vi "CSM-TagDBDisplayWnd.vi"(7 "Name(\"\" to use uuid)":string="UI.Exp.Template") -> ()   [LabVIEW 2020, in "CSM-TagDBDisplayWnd.lvlib"]
doc: "------------- lvcsm -------------\n[CSMStates]\nItem 0 = \"Idle\"\nItem 1 = \"CSM Documentation\"\nItem 2 = \"VI Reference\"\nItem 3 = \"Error Handler\"\nItem 4 = \"Critical Error\"\nItem 5 = \"Target Timeout Error\"\nItem 6 = \"Target Error\"\nItem 7 = \"Async Response\"\nItem 8 = \"Response\"\nItem 9 = \"Async Message Posted\"\nItem 10 = \"Initialize Core Data\"\nItem 11 = \"Exit\"\nItem 12 = \"Data: Initialize\"\nItem 13 = \"Data: Update Indicators\"\nItem 14 = \"Data: Load Attributes\"\nItem 15 = \"Data: Save Attributes\"\nItem 16 = \"Data: Cleanup\"\nItem 17 = \"Macro: Initialize\"\nItem 18 = \"Macro: Exit\"\nItem 19 = \"API: Start Refreshing\"\nItem 20 = \"API: Stop Refreshing\"\nItem 21 = \"Action: Insert TestStandOI\"\nItem 22 = \"Action: Relocate Boolean Switchs\"\nItem 23 = \"Action: Refresh Check\"\n\n[CSMStatus]\nItem 0 = \"Error Occurred@Error Handler\""
uses:
  CSM-TagDBDisplayWnd.lvlib
  a2febdbb-fb03-4ba6-9898-8a5d1d02332c.vi
  254342f9-cc88-4ec7-9cbe-7727ec765c53.vi
  d50deaec-bb00-4691-9d91-a2e409c005f3.vi
  1aa7de20-dba2-4569-9d21-b3d571cae75a.vi
  cbb8679f-6fca-4dfa-96de-e02d92bb6012.vi
  <userlib>/_NEVSTOP/Communicable State Machine(CSM)/AdvanceAPI/CSM - Revert Arguments-Safe String.vi
  <userlib>/_NEVSTOP/Communicable State Machine(CSM)/_Shared/Trim Single-line Text.vi
  <userlib>/_NEVSTOP/Communicable State Machine(CSM)/AdvanceAPI/CSM - Make String Arguments Safe.vi
  <userlib>/_NEVSTOP/Communicable State Machine(CSM)/AdvanceAPI/CSM - Break Down Multiple States String.vi
  <userlib>/_NEVSTOP/Communicable State Machine(CSM)/AdvanceAPI/CSM - Compact Multiple States.vi
  a2febdbb-fb03-4ba6-9898-8a5d1d02332c.vi/99de0c97-112a-4c86-9094-c187659127e1.vi
  <userlib>/_NEVSTOP/Communicable State Machine(CSM)/Utility/Build Error Cluster.vi
  <userlib>/_NEVSTOP/Communicable State Machine(CSM)/AdvanceAPI/CSM - Convert HexStr to Data.vi
  <userlib>/_NEVSTOP/Communicable State Machine(CSM)/AdvanceAPI/CSM - Keywords.vi
  <userlib>/_NEVSTOP/Communicable State Machine(CSM)/_Polymophic/CSM - Filter Duplicated Lines.vi
  <vilib>/Utility/Data Type/Get Type Information.vi
  <userlib>/_NEVSTOP/Communicable State Machine(CSM)/addons/API-String-Arugments-Support/_Support/Data To SingleElementsArray_csm.vi
  <userlib>/_NEVSTOP/Communicable State Machine(CSM)/addons/API-String-Arugments-Support/_Support/Data To API String Arguments.vi
  <userlib>/_NEVSTOP/Communicable State Machine(CSM)/addons/INI-Static-Variable-Support/_Support/Parse Used Session and Name.vi
  <userlib>/_NEVSTOP/Communicable State Machine(CSM)/addons/INI-Static-Variable-Support/_Support/INI-FGV(lvlibp).vi
  <userlib>/_NEVSTOP/Communicable State Machine(CSM)/addons/INI-Static-Variable-Support/_Support/Populate String with INI Variable.vi
  <userlib>/_NEVSTOP/Communicable State Machine(CSM)/addons/API-String-Arugments-Support/_Support/Convert API String Arguments to Data(variant).vi
  <userlib>/_NEVSTOP/Communicable State Machine(CSM)/addons/API-String-Arugments-Support/_Support/SingleElementsArray To Data_csm.vi
  <userlib>/_NEVSTOP/TagDB/Add-ons/RefManager/_Support/UISync/_Pull Controls Value to DPs(VI).vi
  <userlib>/_NEVSTOP/TagDB/Add-ons/RefManager/_Support/UISync/_Publish DP Indicators(VI).vi
  DefaultPage.vi
  <userlib>/_NEVSTOP/Communicable State Machine(CSM)/Communicable State Machine.lvlib
  <userlib>/_NEVSTOP/Communicable State Machine(CSM)/addons/Logger/CSM File Logger.lvlib
  <userlib>/_NEVSTOP/Communicable State Machine(CSM)/addons/Loop-Support/CSM Loop Support.lvlib
  <userlib>/_NEVSTOP/Communicable State Machine(CSM)/addons/INI-Static-Variable-Support/INI-Static-Variable-Support.lvlib
  <userlib>/_NEVSTOP/TagDB/TagDB.lvlib
  <userlib>/_NEVSTOP/TagDB/Add-ons/RefManager/TagDB RefManager.lvlib
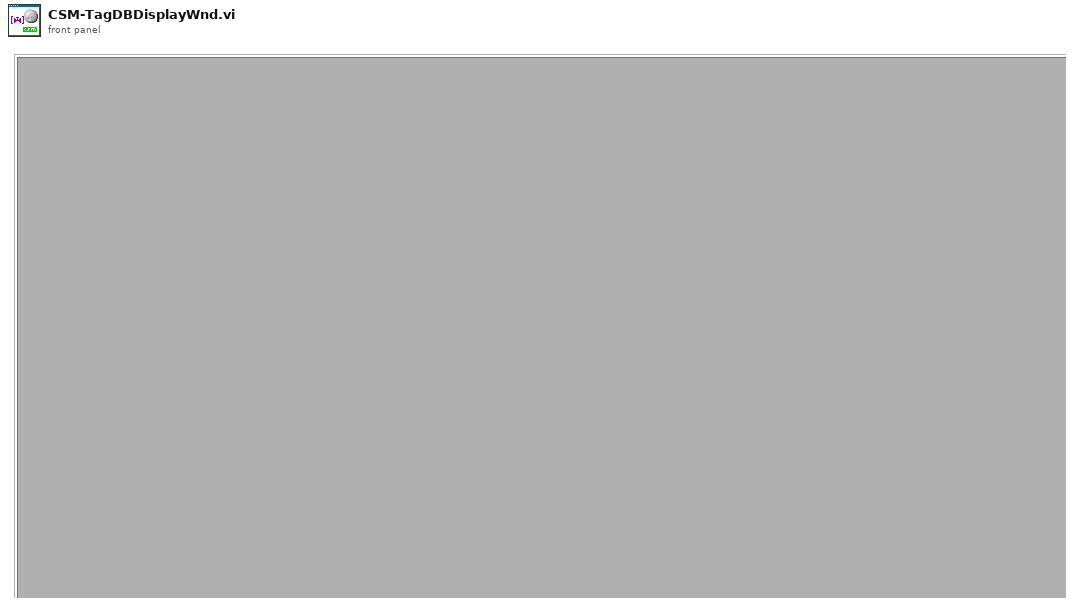
[diagram p1: front panel]
types:
  T1 = enum32{"Invalid", "Standard", "Closed", "Hidden", "Minimized", "Maximized"}
  T2 = enum32{"invalid app kind", "Development System", "Run Time System", "Student Edition", "Embedded LabVIEW", "Evaluation", "Custom"}
  T3 = typedef "Communicable State Machine.lvlib/_CSM_Response Source Message.ctl" = cluster{"‘State":string, "’Arguments":string, "’Error":errorcluster}
  T4 = cluster{"Current VI Reference":refnum<vi>, "Close Panel on Exit?":bool}
  T5 = cluster{"Core":cluster{"Current VI Reference":refnum<vi>, "Close Panel on Exit?":bool}, "SearchingPath":path[], "PageRef":refnum<vi>, "DefaultPage":string}
  T6 = cluster{"SearchingPath":path[], "DefaultPage":string}
  T7 = enum32{"Bad", "Idle", "Run top level", "Running"}
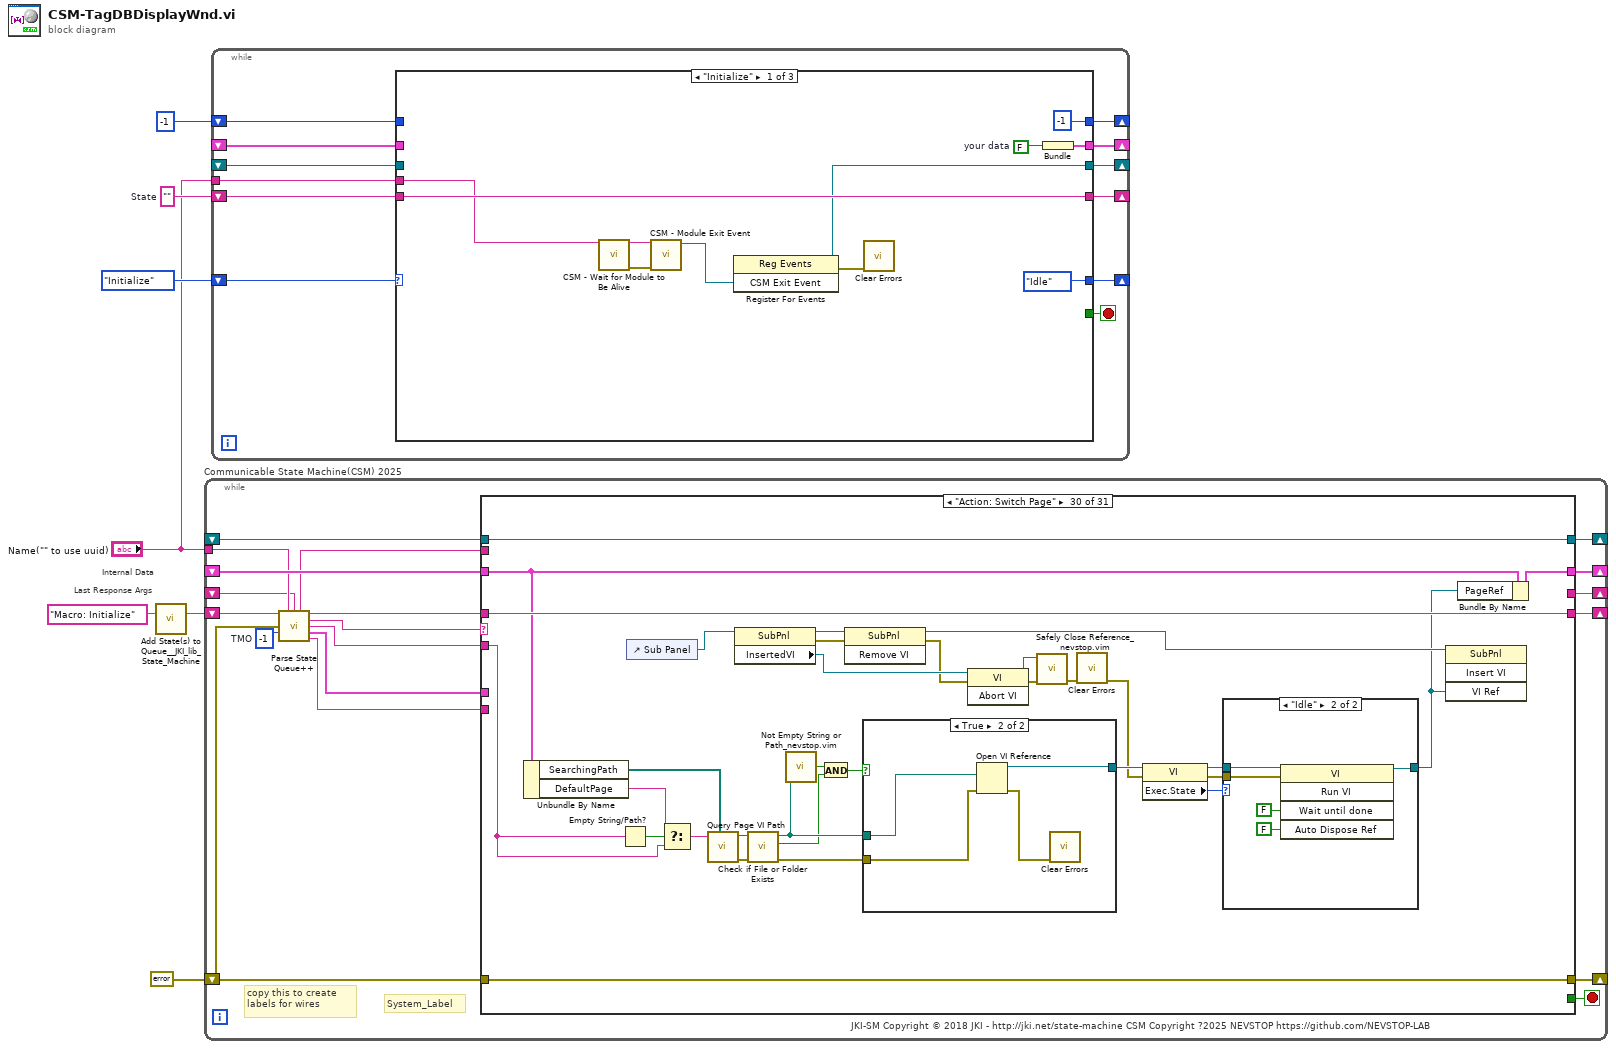
[diagram p0: block diagram]
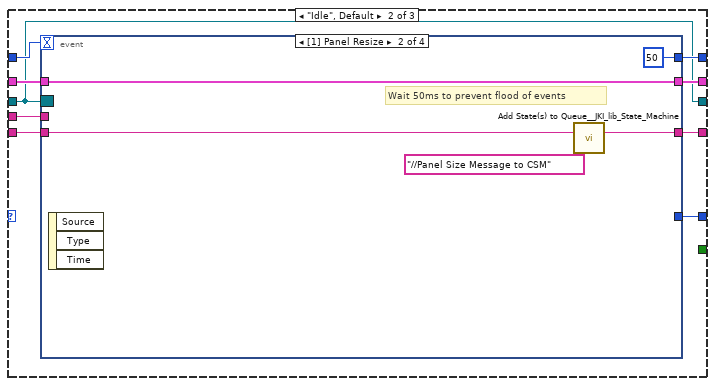
[diagram p2: hidden frame]
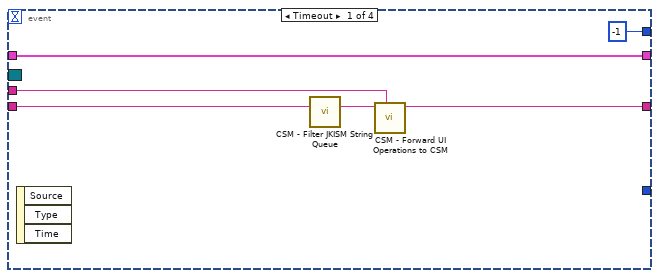
[diagram p3: hidden frame]
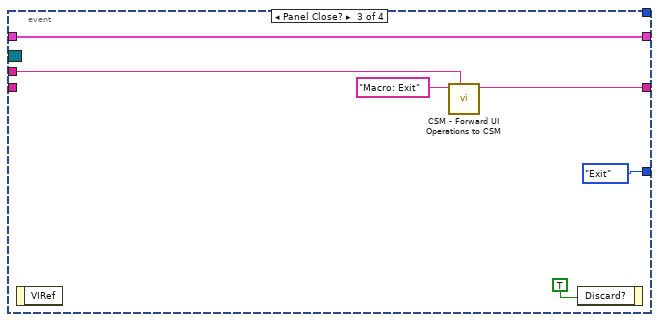
[diagram p4: hidden frame]
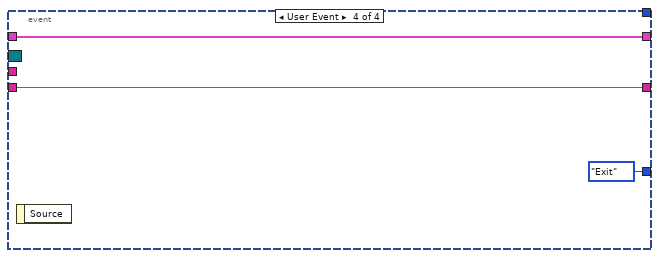
[diagram p5: hidden frame]
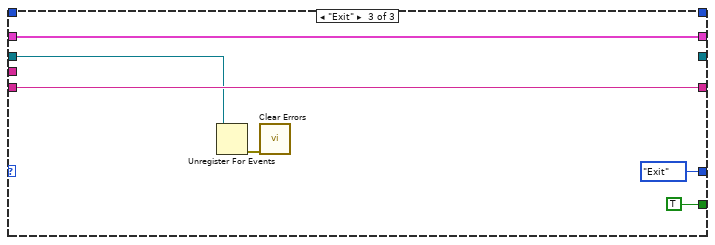
[diagram p6: hidden frame]
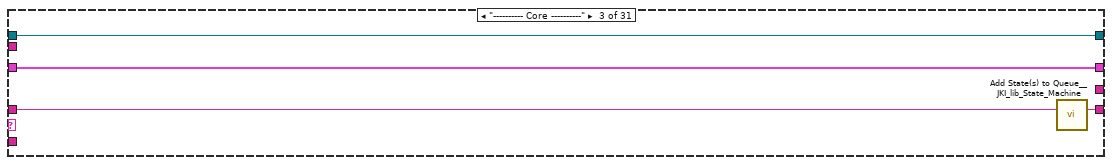
[diagram p9: hidden frame]
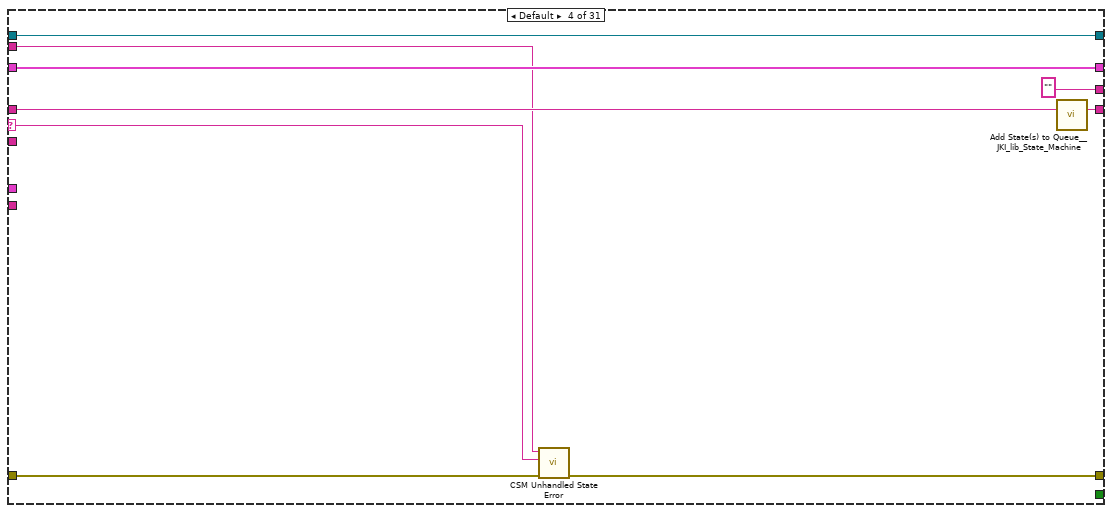
[diagram p10: hidden frame]
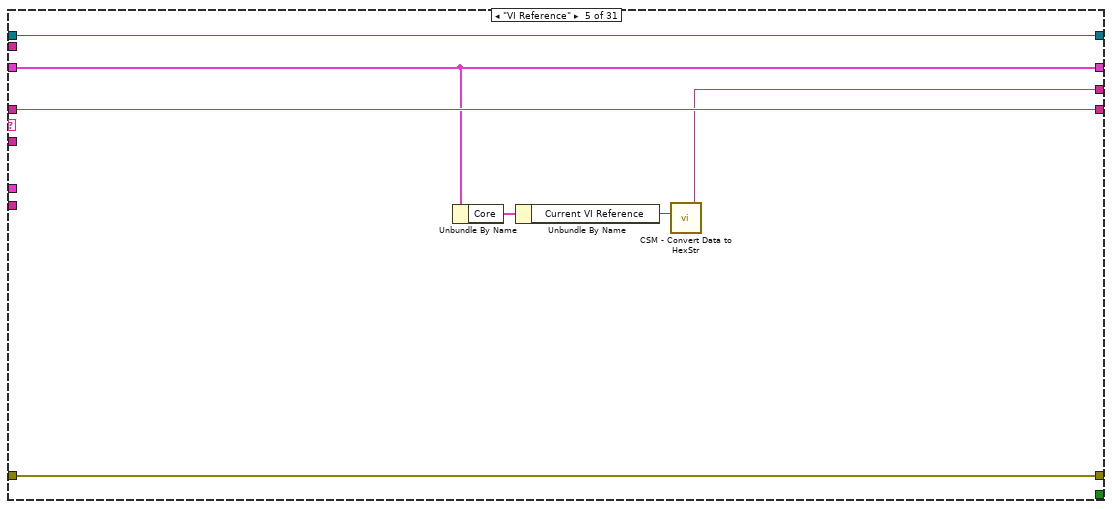
[diagram p11: hidden frame]
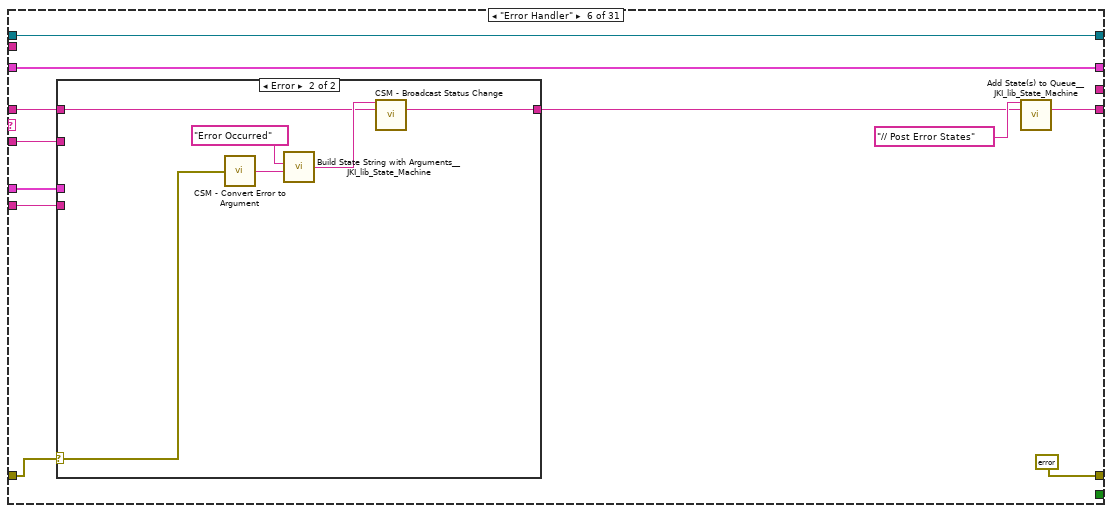
[diagram p12: hidden frame]
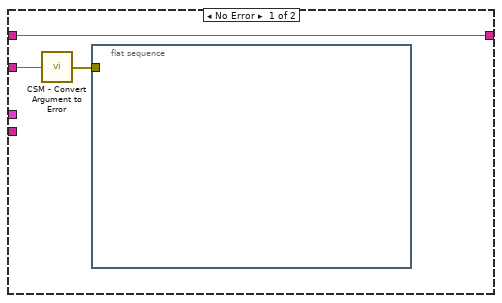
[diagram p13: hidden frame]
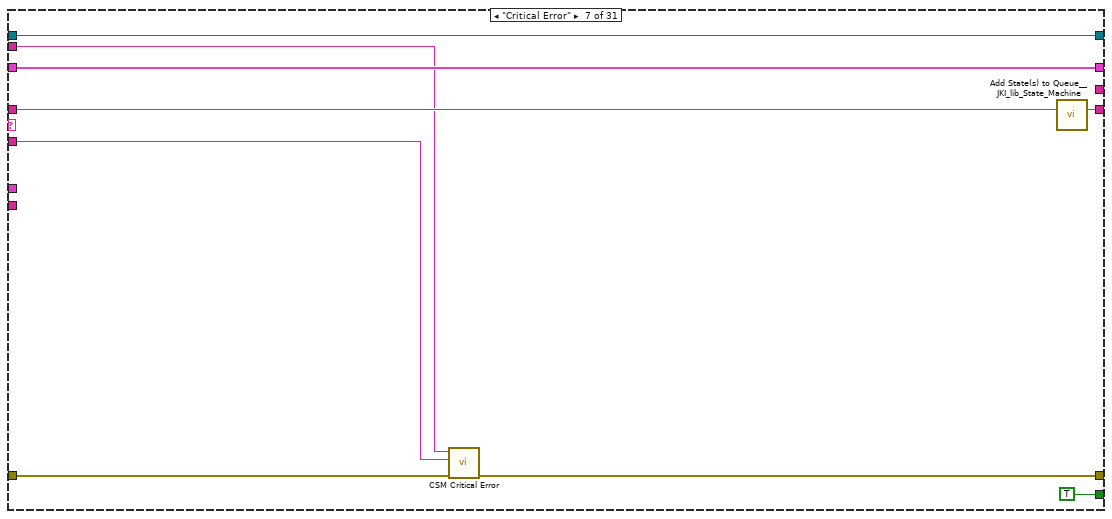
[diagram p14: hidden frame]
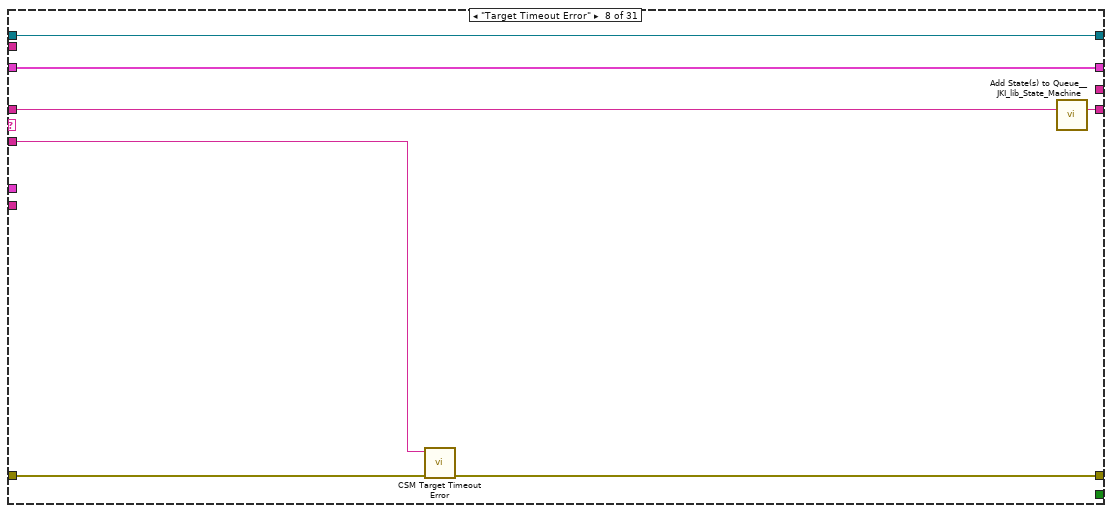
[diagram p15: hidden frame]
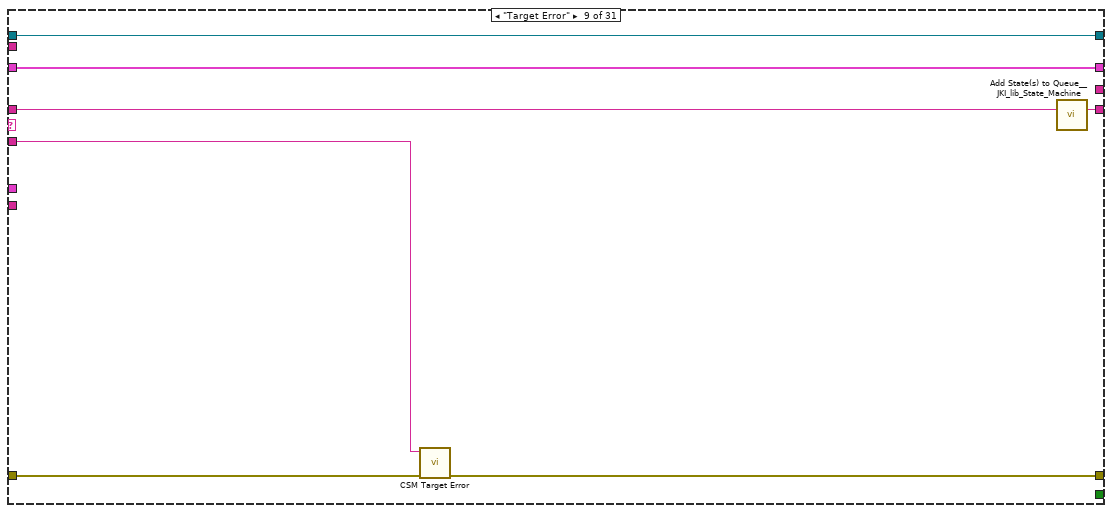
[diagram p16: hidden frame]
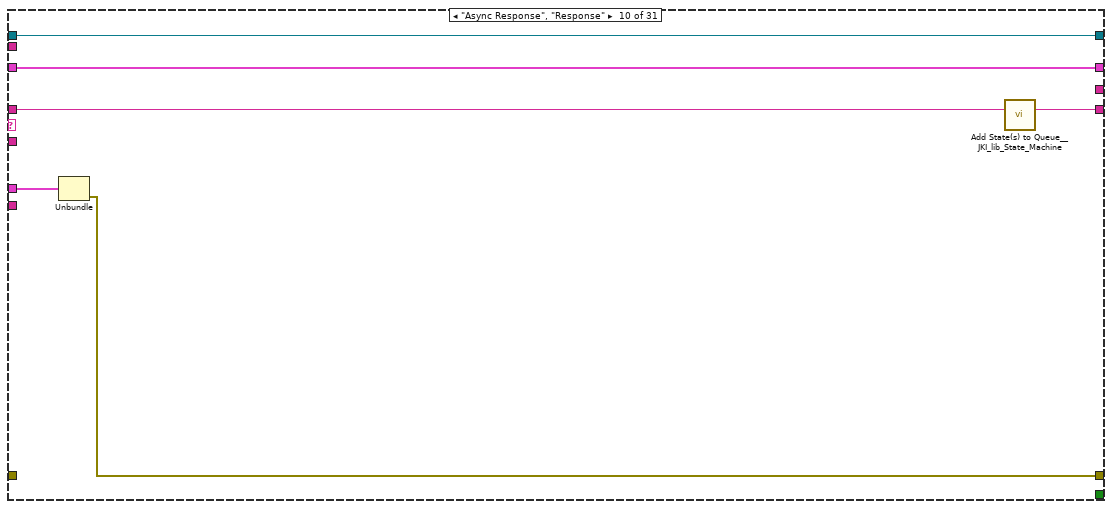
[diagram p17: hidden frame]
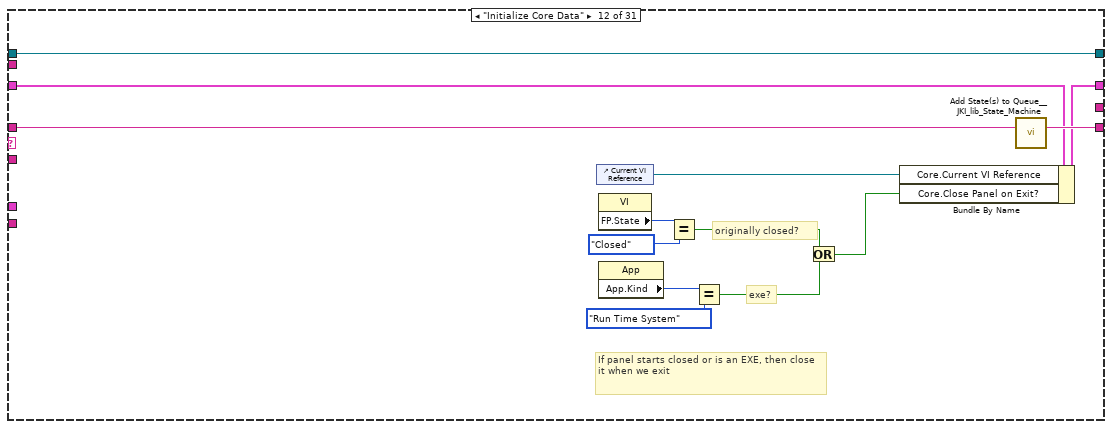
[diagram p19: hidden frame]
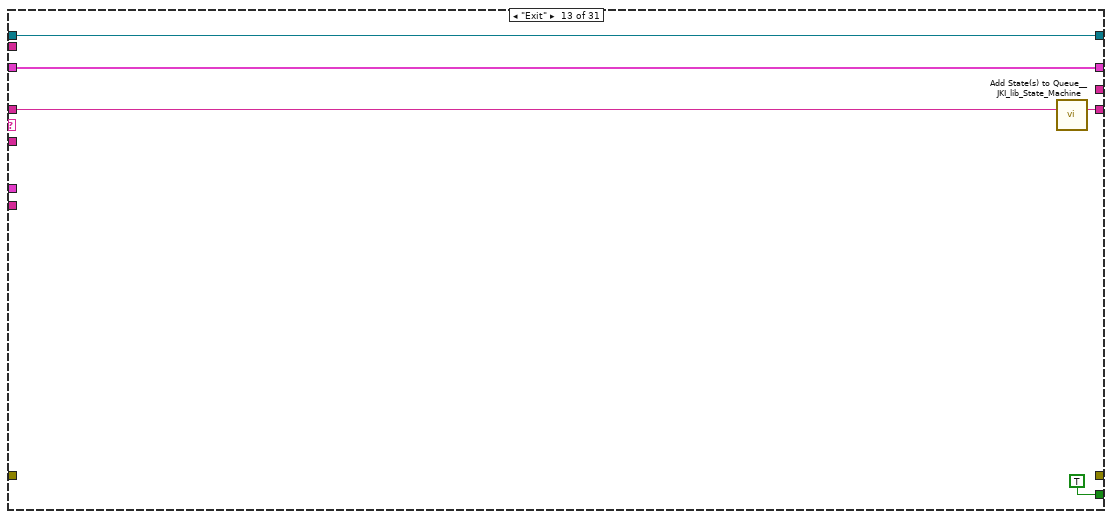
[diagram p20: hidden frame]
diagram:
  w3 = ""  # State
  # "Last Response Args"
  # "Internal Data"
  n1 = call <vilib>:"Add State(s) to Queue__JKI_lib_State_Machine.vi"("State(s) in (\"\")"="Macro: Initialize" ("Init State(\"Macro: Initialize\")")) -> ("States Out"=w7:string)  [unwired: 14 in]
  n2 = while "Communicable State Machine(CSM) 2025" {
    shift-right: [w21] -> _
    shift-left: _ -> [w20]
    shift-right: [w24] -> _
    shift-left: errorcluster {"status"=FALSE, "code"=0, "source"=""} ("error out") -> [w10]
    shift-right: [w23] -> _
    shift-left: w7 -> [w25]
    tunnel: "Name(\"\" to use uuid)" -> [w17]
    shift-right: [w18] -> _
    shift-left: _ -> [w12]
    shift-right: [w9] -> _
    shift-left: _ -> [w8]
    stop <- w22 stop-if-true
    w19 = -1  # TMO
    # "JKI-SM Copyright © 2018 JKI - http://jki.net/state-machine CSM Copyright ?2025 NEVSTOP https://github.com/NEVSTOP-LAB"
    # "copy this to create labels for wires"
    # "System_Label"
    n3 = call <userlib>:"Parse State Queue++.vi"("State Queue"=w25, "Name (\"\" to Use UUID)"=w17, "Response Arguments"=w12, "Previous Error"=w10, "Dequeue (1 ms)"=w19) -> ("Name Used"=w11:string, "Remaining States"=w26:string, "Current State"=w13:string, "Arguments"=w14:string, "Additional Information"=w15:T3, "Source CSM"=w16:string)  [unwired: 5 in]
    n4 = case shown="\"Action: Switch Page\"" w13 {
      selector: w13 -> [_ _ _ w41 _ _ _ _ _ _ _ _ _ _ _ _ _ _ _ _ _ _ _ _ _ _ _ _ _ _ w289]
      tunnel: w26 -> [w28 w32 w36 w45 w51 w57 w81 w88 w95 w101 w104 w117 w122 w126 w147 w150 w153 w156 w171 w175 w180 w187 w190 w198 w209 w216 w222 w226 w235 w275 w292]
      tunnel: w14 -> [_ _ _ _ _ w56 w77 w85 w92 _ _ _ _ _ _ _ _ _ _ _ _ _ _ w193 w206 _ _ _ _ w262 _]
      tunnel: w20 -> [w29 w31 w34 w43 w50 w62 w79 w86 w93 w99 w103 w111 w120 w124 _ w149 w152 w155 w166 w173 w178 w185 w189 w197 w212 w218 w221 w224 w232 w269 w294]
      tunnel: [_ _ _ w38 w52 errorcluster {"status"=FALSE, "code"=0, "source"=""} ("error out") w74 w83 w90 w97 _ _ _ _ w133 _ _ _ w167 _ _ _ _ w194 w213 _ _ _ w227 w276 w295] -> w24
      tunnel: w10 -> [_ _ _ w39 w52 w60 w75 w84 w91 _ _ _ _ _ _ _ _ _ w168 _ _ _ _ _ w213 _ _ _ w228 w276 w295]
      tunnel: [w28 w32 w35 w44 w51 w58 w80 w87 w94 w100 w104 w116 w121 w125 w146 w150 w153 w156 w170 w174 w179 w186 w190 w198 w210 w215 w219 w225 w235 w275 w291] -> w23
      tunnel: [_ _ _ _ _ _ TRUE _ _ _ _ _ TRUE _ _ _ _ _ _ _ _ _ _ _ _ _ _ _ _ _ _] -> w22
      tunnel: [w29 w31 w34 w43 w50 w62 w79 w86 w93 w99 w103 w115 w120 w124 w138 w149 w152 w155 w166 w173 w178 w185 w189 w197 w212 w218 w221 w224 w232 w246 w294] -> w21
      tunnel: w16 -> [_ _ _ _ _ w55 _ _ _ _ _ _ _ _ _ _ _ _ _ _ _ _ _ _ _ _ _ _ _ _ _]
      tunnel: w15 -> [_ _ _ _ _ w54 _ _ _ w98 _ _ _ _ _ _ _ _ _ _ _ _ _ _ _ _ _ _ _ _ _]
      tunnel: [_ _ _ "" w47 _ _ _ _ _ _ _ _ _ _ _ _ _ _ _ _ _ _ _ _ _ _ _ _ _ _] -> w18
      tunnel: w11 -> [_ _ _ w40 _ _ w76 _ _ _ _ _ _ _ w140 _ _ _ _ _ _ _ _ _ _ _ _ _ _ _ _]
      tunnel: [w27 w30 w33 w37 w46 w53 w73 w82 w89 w96 w102 w105 w118 w123 refnum<k1> refnum ("TagDB") w148 w151 w154 w165 w172 w176 w181 w188 w195 w211 w217 w220 w223 w233 w274 w293] -> w9
      tunnel: w8 -> [w27 w30 w33 w37 w46 w53 w73 w82 w89 w96 w102 w105 w118 w123 _ w148 w151 w154 w165 w172 w176 w181 w188 w196 w211 w217 w220 w223 w234 w274 w293]
      frame "", "Idle" {
      }
      frame "CSM Documentation" {
      }
      frame "---------- Core ----------" {
        n5 = call <vilib>:"Add State(s) to Queue__JKI_lib_State_Machine.vi"("State(s) in (\"\")"=w36) -> ("States Out"=w35:string)  [unwired: 14 in]
      }
      frame Default {
        n6 = call <userlib>:"CSM Unhandled State Error.vi"("error in (no error)"=w39, "Undefined State"=w41, "CSM Name"=w40) -> ("error out"=w38:errorcluster)  [unwired: 8 in]
        n7 = call <vilib>:"Add State(s) to Queue__JKI_lib_State_Machine.vi"("State(s) in (\"\")"=w45) -> ("States Out"=w44:string)  [unwired: 14 in]
      }
      frame "VI Reference" {
        n8 = Unbundle By Name(w50) -> ("Core"=w49:T4)
        n9 = Unbundle By Name(w49) -> ("Current VI Reference"=w48:refnum<vi>)
        n10 = call <userlib>:"CSM - Convert Data to HexStr.vi"("Variant"=w48) -> ("HEX String (0-9,A-F)"=w47:string)  [unwired: 8 in]
      }
      frame "Error Handler" {
        n11 = case shown="Error" w60 {
          selector: w60 -> [_ w67]
          tunnel: [w66 w69] -> w59
          tunnel: w57 -> [w66 w68]
          tunnel: w56 -> [w65 _]
          tunnel: w55 -> [_ _]
          tunnel: w54 -> [_ _]
          frame No Error {
            n12 = call <userlib>:"CSM - Convert Argument to Error.vi"("Argument"=w65) -> ("Error"=w64:errorcluster)  [unwired: 4 in]
            n13 = flat-sequence {
              tunnel: w64 -> [_]
              frame #0 {
              }
            }
          }
          frame Error {
            n14 = call <userlib>:"CSM - Convert Error to Argument.vi"("Error"=w67) -> ("Argument"=w71:string)  [unwired: 4 in]
            n15 = call <vilib>:"Build State String with Arguments__JKI_lib_State_Machine.vi"("Arguments (\"\")"=w71, "State"="Error Occurred" ("Status with Arguments")) -> ("State with Arguments"=w70:string)  [unwired: 4 in]
            n16 = call <userlib>:"CSM - Broadcast Status Change.vi"("Status With Arguments"=w70, "State Queue"=w68) -> ("Remaining States"=w69:string)  [unwired: 13 in]
          }
        }
        n17 = call <vilib>:"Add State(s) to Queue__JKI_lib_State_Machine.vi"("State(s) in Front (\"\")"="// Post Error States", "State(s) in (\"\")"=w59) -> ("States Out"=w58:string)  [unwired: 13 in]
      }
      frame "Critical Error" {
        n18 = call <userlib>:"CSM Critical Error.vi"("error in (no error)"=w75, "Arugments (As Reason)"=w77, "CSM Name"=w76) -> ("error out"=w74:errorcluster)  [unwired: 8 in]
        n19 = call <vilib>:"Add State(s) to Queue__JKI_lib_State_Machine.vi"("State(s) in (\"\")"=w81) -> ("States Out"=w80:string)  [unwired: 14 in]
      }
      frame "Target Timeout Error" {
        n20 = call <userlib>:"CSM Target Timeout Error.vi"("error in (no error)"=w84, "Arguments (As CSM Name)"=w85) -> ("error out"=w83:errorcluster)  [unwired: 9 in]
        n21 = call <vilib>:"Add State(s) to Queue__JKI_lib_State_Machine.vi"("State(s) in (\"\")"=w88) -> ("States Out"=w87:string)  [unwired: 14 in]
      }
      frame "Target Error" {
        n22 = call <userlib>:"CSM Target Error.vi"("error in (no error)"=w91, "Arguments (As CSM Name)"=w92) -> ("error out"=w90:errorcluster)  [unwired: 9 in]
        n23 = call <vilib>:"Add State(s) to Queue__JKI_lib_State_Machine.vi"("State(s) in (\"\")"=w95) -> ("States Out"=w94:string)  [unwired: 14 in]
      }
      frame "Async Response", "Response" {
        n24 = Unbundle(w98) -> ("’Error"=w97:errorcluster)  [unwired: 2 out]
        n25 = call <vilib>:"Add State(s) to Queue__JKI_lib_State_Machine.vi"("State(s) in (\"\")"=w101) -> ("States Out"=w100:string)  [unwired: 14 in]
      }
      frame "Async Message Posted" {
      }
      frame "Initialize Core Data" {
        # "originally closed?"
        # "exe?"
        # "If panel starts closed or is an EXE, then close it when we exit"
        n26 = control-ref of="Current VI Reference"() -> (w109:refnum<vi>)
        n27 = property class="VI"() -> ("FP.State"=w108:T1)  [unwired: 2 in, 2 out]
        n28 = property class="App"() -> ("App.Kind"=w114:T2)  [unwired: 2 in, 2 out]
        n29 = Equal?(x=w108, y=T1."Closed" ("Front Panel Window:State")) -> (x = y?=w106:bool)
        n30 = Equal?(x=w114, y=T2."Run Time System" ("Application:Kind")) -> (x = y?=w112:bool)
        n31 = Or(x=w106, y=w112) -> (x .or. y?=w110:bool)
        n32 = Bundle By Name(cluster=w111, "Core.Current VI Reference"=w109, "Core.Close Panel on Exit?"=w110) -> (w115:T5)
        n33 = call <vilib>:"Add State(s) to Queue__JKI_lib_State_Machine.vi"("State(s) in (\"\")"=w117) -> ("States Out"=w116:string)  [unwired: 14 in]
      }
      frame "Exit" {
        n34 = call <vilib>:"Add State(s) to Queue__JKI_lib_State_Machine.vi"("State(s) in (\"\")"=w122) -> ("States Out"=w121:string)  [unwired: 14 in]
      }
      frame "---------- Data ----------" {
        n35 = call <vilib>:"Add State(s) to Queue__JKI_lib_State_Machine.vi"("State(s) in (\"\")"=w126) -> ("States Out"=w125:string)  [unwired: 14 in]
      }
      frame "Data: Initialize" {
        w127 = "*"  # DefaultPage
        w137 = ""  # DefaultPage
        w142 = refnum<vi> refnum  # PageRef
        w139 = path[] []  # SearchingPath
        w144 = T4 {"Current VI Reference"=refnum, "Close Panel on Exit?"=FALSE}  # Core
        n36 = Bundle("Core"=w144, "SearchingPath"=w139, "PageRef"=w142, "DefaultPage"=w137) -> (w145:T5)  [unwired: 1 in]
        n37 = Bundle("SearchingPath"=w139, "DefaultPage"=w137) -> (w141:T6)  [unwired: 1 in]
        n38 = call "CSM - Read Cluster Elements From Session.vim"("Section Name (\"\" as Default)"=w140, "Cluster"=w141) -> ("error out"=w133:errorcluster, "Cluster out"=w136:T6)  [unwired: 6 in]
        n39 = Unbundle By Name(w136) -> ("SearchingPath"=w135:path[], "DefaultPage"=w134:string)
        n40 = call <userlib>:"CSM Application Directory.vi"() -> ("CSM Application Dir"=w128:path)  [unwired: 11 in]
        n41 = Current VI's Path() -> (path=w131:path)
        n42 = Build Path(base path=w128, name or relative path=w127) -> (appended path=w129:path)
        n43 = call <userlib>:"First Existing Folder in Path.vi"("Stripped Path In"=w131) -> ("Stripped Path Out"=w130:path)  [unwired: 10 in]
        n44 = Build Array (concatenate)(w135, w130, w129) -> (w132:path[])
        n45 = Bundle By Name(cluster=w145, "SearchingPath"=w132, "DefaultPage"=w134) -> (w138:T5)
        n46 = call <vilib>:"Add State(s) to Queue__JKI_lib_State_Machine.vi"("State(s) in (\"\")"=w147) -> ("States Out"=w146:string)  [unwired: 14 in]
      }
      frame "Data: Update Indicators" {
      }
      frame "Data: Load Attributes" {
      }
      frame "Data: Save Attributes" {
      }
      frame "Data: Cleanup" {
        n47 = Unbundle By Name(w166) -> ("Core.Current VI Reference"=w169:refnum<vi>)
        n48 = control-ref of="Sub Panel"() -> (w164:refnum<vi>)
        n49 = property class="SubPnl"(reference=w164) -> (reference out=w158:refnum<vi>, error out=w159:errorcluster, "InsertedVI"=w163:refnum<vi>)  [unwired: 1 in]
        n50 = invoke class="SubPnl" method="Remove VI"(reference=w158, error in=w159) -> (error out=w157:errorcluster)  [unwired: 1 in, 2 out]
        n51 = Close Reference(reference=w169, error in (no error)=w168) -> (error out=w167:errorcluster)
        n52 = invoke class="VI" method="Abort VI"(reference=w163, error in=w157) -> (reference out=w161:refnum<vi>, error out=w162:errorcluster)  [unwired: 1 in, 1 out]
        n53 = call "Safely Close Reference_nevstop.vim"("error in (no error)"=w162, "Reference"=w161) -> ("error out"=w160:errorcluster)  [unwired: 9 in]
        n54 = call <vilib>:"Clear Errors.vi"("error in (no error)"=w160) -> ()  [unwired: 5 in, 2 out]
        n55 = call <vilib>:"Add State(s) to Queue__JKI_lib_State_Machine.vi"("State(s) in (\"\")"=w171) -> ("States Out"=w170:string)  [unwired: 14 in]
      }
      frame "---------- Macro ----------" {
        n56 = call <vilib>:"Add State(s) to Queue__JKI_lib_State_Machine.vi"("State(s) in (\"\")"=w175) -> ("States Out"=w174:string)  [unwired: 14 in]
      }
      frame "Macro: Initialize" {
        n57 = call <vilib>:"Add State(s) to Queue__JKI_lib_State_Machine.vi"("State(s) in Front (\"\")"="Data: Initialize\nData: Load Attributes\nInitialize Core Data\nData: Update Indicators\nAction: Switch Page\nAPI: Start", "State(s) in (\"\")"=w180) -> ("States Out"=w179:string)  [unwired: 13 in]
      }
      frame "Macro: Exit" {
        n58 = call <vilib>:"Add State(s) to Queue__JKI_lib_State_Machine.vi"("State(s) in Front (\"\")"="//Exit Sub-Modules ", "State(s) at Back (\"\")"="Data: Save Attributes\nData: Cleanup\nExit") -> ("States Out"=w183:string)  [unwired: 13 in]
        n59 = call <vilib>:"Add State(s) to Queue__JKI_lib_State_Machine.vi"("State(s) in Front (\"\")"=w183, "State(s) in (\"\")"=w187) -> ("States Out"=w186:string)  [unwired: 13 in]
      }
      frame "---------- API ----------" {
      }
      frame "API: Set TagDB" {
        n60 = call <userlib>:"Is HexStr Content.vi"("Content"=w193) -> ("hexStr"=w191:string, "HexStr Content"=w192:bool)  [unwired: 9 in]
        n61 = case shown="True" w192 {
          tunnel: w196 -> [_ w205]
          tunnel: [w201 w204] -> w195
          tunnel: [w200 w203] -> w194
          tunnel: w191 -> [w199 w202]
          frame False {
            n62 = call <userlib>:"TagDB-Obtain.vi"("name (unnamed)"=w199) -> ("error out"=w200:errorcluster, "TagDB"=w201:refnum<k1>)  [unwired: 4 in, 1 out]
          }
          frame True {
            n63 = call "CSM - Convert HexStr to Data.vim"("Type"=w205, "HEX String"=w202) -> ("Error out"=w203:errorcluster, "data"=w204:refnum<k1>)  [unwired: 6 in]
          }
        }
      }
      frame "API: Switch" {
        n64 = call <vilib>:"Build State String with Arguments__JKI_lib_State_Machine.vi"("Arguments (\"\")"=w206, "State"="Action: Switch Page") -> ("State with Arguments"=w207:string)  [unwired: 4 in]
        n65 = call <vilib>:"Add State(s) to Queue__jki_lib_state_machine.vi"("State(s) in Front (\"\")"=w207, "State(s) in (\"\")"=w209) -> ("States Out"=w210:string)  [unwired: 13 in]
      }
      frame "API: Start" {
        n66 = call <userlib>:"CSMLS - Define Loop State(s).vi"("Loop States"="Action: Loop Check -><loop>", "States Queue"=w216) -> ("Remaining States"=w215:string)  [unwired: 13 in]
      }
      frame "API: Stop" {
        n67 = call <userlib>:"CSMLS - Remove Loop Tag to Break.vi"("States Queue"=w222) -> ("Remaining States"=w219:string)  [unwired: 10 in]
      }
      frame "---------- Action ----------" {
        n68 = call <vilib>:"Add State(s) to Queue__JKI_lib_State_Machine.vi"("State(s) in (\"\")"=w226) -> ("States Out"=w225:string)  [unwired: 14 in]
      }
      frame "Action: Refresh TagDB Display" {
        n69 = Unbundle By Name(w232) -> ("PageRef"=w231:refnum<vi>)
        n70 = Not A Number/Path/Refnum?(number/path/refnum=w231) -> (NaN/Path/Refnum?=w229:bool)
        n71 = Not(x=w229) -> (.not. x?=w230:bool)
        n72 = case shown="True" w230 {
          tunnel: w234 -> [w237 w244]
          tunnel: [w237 w242] -> w233
          tunnel: w231 -> [_ w238]
          tunnel: w228 -> [w236 w239]
          tunnel: [w236 w241] -> w227
          frame False {
          }
          frame True {
            n73 = call-poly <userlib>:"Pull Controls Value to DPs.vi"("VIRef(Caller VI)"=w238, "error in (no error)"=w239, "SILAPI In"=w244) -> ("error out"=w240:errorcluster, "SILAPI Out"=w243:refnum<k1>)  [unwired: 6 in, 1 out]
            n74 = call-poly <userlib>:"Publish DP Indicators.vi"("VIRef(Caller VI)/RefMgr"=w238, "error in (no error)"=w240, "SILAPI In"=w243) -> ("error out"=w241:errorcluster, "SILAPI Out"=w242:refnum<k1>)  [unwired: 6 in, 1 out]
          }
        }
      }
      frame "Action: Switch Page" {
        n75 = Unbundle By Name(w269) -> ("SearchingPath"=w268:path[], "DefaultPage"=w263:string)
        n76 = Empty String/Path?(string/path=w262) -> (empty?=w264:bool)
        n77 = control-ref of="Sub Panel"() -> (w249:refnum<vi>)
        n78 = Select(t=w263, s=w264, f=w262) -> (s? t:f=w261:string)
        n79 = call "Query Page VI Path.vi"("searching path"=w268, "page name"=w261) -> ("Error out"=w266:errorcluster, "path"=w267:path)  [unwired: 8 in]
        n80 = property class="SubPnl"(reference=w249) -> (reference out=w251:refnum<vi>, error out=w252:errorcluster, "InsertedVI"=w256:refnum<vi>)  [unwired: 1 in]
        n81 = call <vilib>:"Check if File or Folder Exists.vi"("error in (no error)"=w266, "path"=w267) -> ("error out"=w265:errorcluster, "file or folder exists?"=w258:bool, "dup path"=w260:path)  [unwired: 7 in]
        n82 = call "Not Empty String or Path_nevstop.vim"("String"=w260) -> ("not empty?"=w259:bool)
        n83 = And(x=w259, y=w258) -> (x .and. y?=w257:bool)
        n84 = invoke class="SubPnl" method="Remove VI"(reference=w251, error in=w252) -> (reference out=w247:refnum<vi>, error out=w250:errorcluster)  [unwired: 1 in, 1 out]
        n85 = case shown="True" w257 {
          tunnel: [w277 w281] -> w273
          tunnel: w260 -> [_ w280]
          tunnel: w265 -> [_ w279]
          frame False {
            n86 = vi-ref "CSM-TagDBDisplayWnd.lvlib:DefaultPage.vi"() -> (w277:refnum<vi>)
          }
          frame True {
            n87 = Open VI Reference(vi path=w280, error in (no error)=w279) -> (vi reference=w281:refnum<vi>, error out=w278:errorcluster)  [unwired: 4 in]
            n88 = call <vilib>:"Clear Errors.vi"("error in (no error)"=w278) -> ()  [unwired: 5 in, 2 out]
          }
        }
        n89 = invoke class="VI" method="Abort VI"(reference=w256, error in=w250) -> (reference out=w254:refnum<vi>, error out=w255:errorcluster)  [unwired: 1 in, 1 out]
        n90 = call "Safely Close Reference_nevstop.vim"("error in (no error)"=w255, "Reference"=w254) -> ("error out"=w253:errorcluster)  [unwired: 9 in]
        n91 = call <vilib>:"Clear Errors.vi"("error in (no error)"=w253) -> ("error out"=w248:errorcluster)  [unwired: 5 in, 1 out]
        n92 = property class="VI"(reference=w273, error in=w248) -> (reference out=w272:refnum<vi>, error out=w270:errorcluster, "Exec.State"=w271:T7)
        n93 = case shown="\"Idle\"" w271 {
          tunnel: w272 -> [w282 w285]
          tunnel: [w282 w283] -> w245
          tunnel: w270 -> [_ w284]
          frame "Bad", Default {
          }
          frame "Idle" {
            n94 = invoke class="VI" method="Run VI"(reference=w285, error in=w284, "Wait until done"=FALSE ("Wait Until Done"), "Auto Dispose Ref"=FALSE ("Auto Dispose Reference")) -> (reference out=w283:refnum<vi>)  [unwired: 1 in, 4 out]
          }
        }
        n95 = invoke on="Invoke Node" class="SubPnl" method="Insert VI"(reference=w247, "VI Ref"=w245) -> ()  [unwired: 2 in, 4 out]
        n96 = Bundle By Name(cluster=w269, "PageRef"=w245) -> (w246:T5)
      }
      frame "Action: Loop Check" {
        n97 = Wait (ms)(milliseconds to wait=u32 100) -> ()  [unwired: 1 out]
        n98 = call <userlib>:"CSMLS - Append Continuous State.vi"("Loop State(s) And Arguments"="Action: Refresh TagDB Display", "Continous State"=w289, "States Queue"=w292) -> ("Remaining States"=w291:string)  [unwired: 8 in]
      }
    }
  }
  n99 = while {
    shift-right: [w306] -> _
    shift-left: enum16{"Idle", "Initialize", "Exit"}."Initialize" -> [w307]
    tunnel: "Name(\"\" to use uuid)" -> [w304]
    shift-right: [w302] -> _
    shift-left: w3 -> [w303]
    shift-right: [w300] -> _
    shift-left: -1 -> [w301]
    shift-right: [w299] -> _
    shift-left: _ -> [w296]
    shift-right: [w298] -> _
    shift-left: _ -> [w297]
    stop <- w305 stop-if-true
    n100 = case shown="\"Initialize\"" w307 {
      tunnel: [enum16{"Idle", "Initialize", "Exit"}."Idle" w327 enum16{"Idle", "Initialize", "Exit"}."Exit"] -> w306
      tunnel: [_ _ TRUE] -> w305
      tunnel: w304 -> [w314 w326 _]
      tunnel: w303 -> [w317 w324 w351]
      tunnel: [w317 w325 w351] -> w302
      tunnel: w301 -> [_ w322 _]
      tunnel: [-1 w323 _] -> w300
      tunnel: [w313 w319 _] -> w299
      tunnel: w296 -> [_ w319 w350]
      tunnel: [w309 w320 w348] -> w298
      tunnel: w297 -> [_ w321 w348]
      frame "Initialize" {
        w310 = FALSE  # your data
        n101 = call <userlib>:"CSM - Wait for Module to Be Alive.vi"("CSM Name"=w314) -> ("CSM Name (Dup)"=w312:string, "error out"=w311:errorcluster)  [unwired: 12 in, 1 out]
        n102 = call <userlib>:"CSM - Module Exit Event.vi"("Error In"=w311, "Name (\"\" to Use UUID) In"=w312) -> ("CSM Exit Event"=w315:refnum<user-event>)  [unwired: 7 in, 2 out]
        n103 = register-events(w315) -> (reference out=w313:refnum<event-registration>, error out=w308:errorcluster)  [unwired: 2 in]
        n104 = call <vilib>:"Clear Errors.vi"("error in (no error)"=w308) -> ()  [unwired: 5 in, 2 out]
        n105 = Bundle("your data"=w310) -> (w309:cluster{"your data":bool})  [unwired: 1 in]
      }
      frame "Idle", Default {
        n106 = event shown="[1] Panel Resize" {
          selector: w319 -> [_ _ _ _]
          dyn-events: _ -> [_ _ _ _]
          timeout: w322 -> [_ _ _ _]
          tunnel: [_ _ enum16{"Idle", "Initialize", "Exit"}."Exit" enum16{"Idle", "Initialize", "Exit"}."Exit"] -> w327
          tunnel: w326 -> [w329 _ w341 _]
          tunnel: w324 -> [w332 w338 _ w347]
          tunnel: [w330 w337 w340 w347] -> w325
          tunnel: [-1 50 _ _] -> w323
          tunnel: w321 -> [w328 w334 w339 w345]
          tunnel: [w328 w334 w339 w345] -> w320
          event Timeout {
            n107 = event-data() -> ()  [unwired: 1 in, 3 out]
            n108 = call-poly <userlib>:"CSM - Filter JKISM String Queue.vi"("States In"=w332) -> ("States Out"=w331:string)  [unwired: 14 in]
            n109 = call <userlib>:"CSM - Forward UI Operations to CSM.vi"("Name (\"\" to Use UUID)"=w329, "State(s) In (\"\")"=w331) -> ("States Out"=w330:string)  [unwired: 8 in, 1 out]
          }
          event Panel Resize {
            # "Wait 50ms to prevent flood of events"
            n110 = event-data() -> ()  [unwired: 1 in, 3 out]
            n111 = call <vilib>:"Add State(s) to Queue__JKI_lib_State_Machine.vi"("State(s) in (\"\")"=w338, "State(s) at Back (\"\")"="//Panel Size Message to CSM" ("State(s) at Back (\"\")")) -> ("States Out"=w337:string)  [unwired: 13 in]
          }
          event Panel Close? {
            n112 = event-data() -> ()  [unwired: 1 in, 1 out]
            n113 = call <userlib>:"CSM - Forward UI Operations to CSM.vi"("Name (\"\" to Use UUID)"=w341, "State(s) In (\"\")"="Macro: Exit" ("State")) -> ("States Out"=w340:string)  [unwired: 8 in, 1 out]
            n114 = event-data("Discard?"=TRUE) -> ()  [unwired: 1 in, 1 out]
          }
          event User Event {
            n115 = event-data() -> ()  [unwired: 1 in, 1 out]
          }
        }
      }
      frame "Exit" {
        n116 = Unregister For Events(event registration refnum=w350) -> (error out=w349:errorcluster)  [unwired: 1 in]
        n117 = call <vilib>:"Clear Errors.vi"("error in (no error)"=w349) -> ()  [unwired: 5 in, 2 out]
      }
    }
  }
